vi "recalibrate gyroscopes from h5.vi"(10 "calibration_block":string, 11 "file":string) -> (1 "function return":i32, 2 "calibration_block out":string, 3 "file out":string)   [LabVIEW 2019, in "apdm.lvlib"]
doc: "APDM_EXPORT int apdm_recalibrate_gyroscopes_from_h5(char *file, uint8_t *calibration_block);"
uses:
  apdm.lvlib
  Lee Lab/CP FES Walking 2018/Code/Working/LabVIEW/apdm.dll
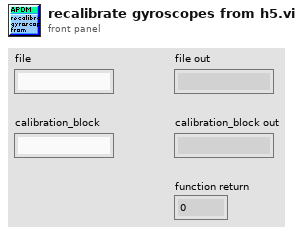
[diagram p1: front panel]
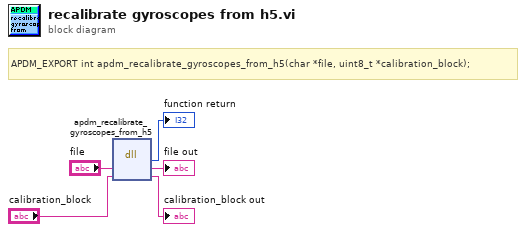
[diagram p0: block diagram]
diagram:
  # "APDM_EXPORT int apdm_recalibrate_gyroscopes_from_h5(char *file, uint8_t *calibration_block);"
  n1 = dll-call lib="C:/Users/jfalesi/Dropbox/Lee Lab/CP FES Walking 2018/Code/Working/LabVIEW/apdm.*" fn="apdm_recalibrate_gyroscopes_from_h5"("file"="file", "calibration_block"="calibration_block") -> (→"function return":i32, "file"=→"file out":string, "calibration_block"=→"calibration_block out":string)  [unwired: 3 in, 2 out]
